vi "主画面.vi"() -> ()   [LabVIEW 2016]
uses:
  <vilib>/Utility/miscctls.llb/LVPointTypeDef.ctl
  <vilib>/ActorFramework/Message Enqueuer/Message Enqueuer.lvclass/Message Enqueuer.ctl
  <vilib>/Utility/miscctls.llb/LVRectTypeDef.ctl
  <vilib>/ActorFramework/Message Enqueuer/Enqueue.vi
  <vilib>/ActorFramework/Stop Msg/Stop Msg.lvclass
  C:/Program Files (x86)/National Instruments/LabVIEW 2016/vi.lib/ActorFramework/Message/Message.lvclass
  <vilib>/ActorFramework/Message Priority Queue/Priority Enqueue.vi
  data/FreeMem.dll
panel:
  out "运行时间":string="运行时间"
  out "ver":string
  out "权限等级 2":enum16{"一级权限", "二级权限", "三级权限", "超级权限"}(ring)
  out "权限等级":string
  out "布尔":bool
  in  "关于":bool
  out "SN":string="SN "
  in  "全屏":T1
  out "站点名称":string="站点名称"
  out "时间显示":string="2017-05-09 10:50:42"
  in  "主画面菜单":T2
  # "水质在线自动监测系统"
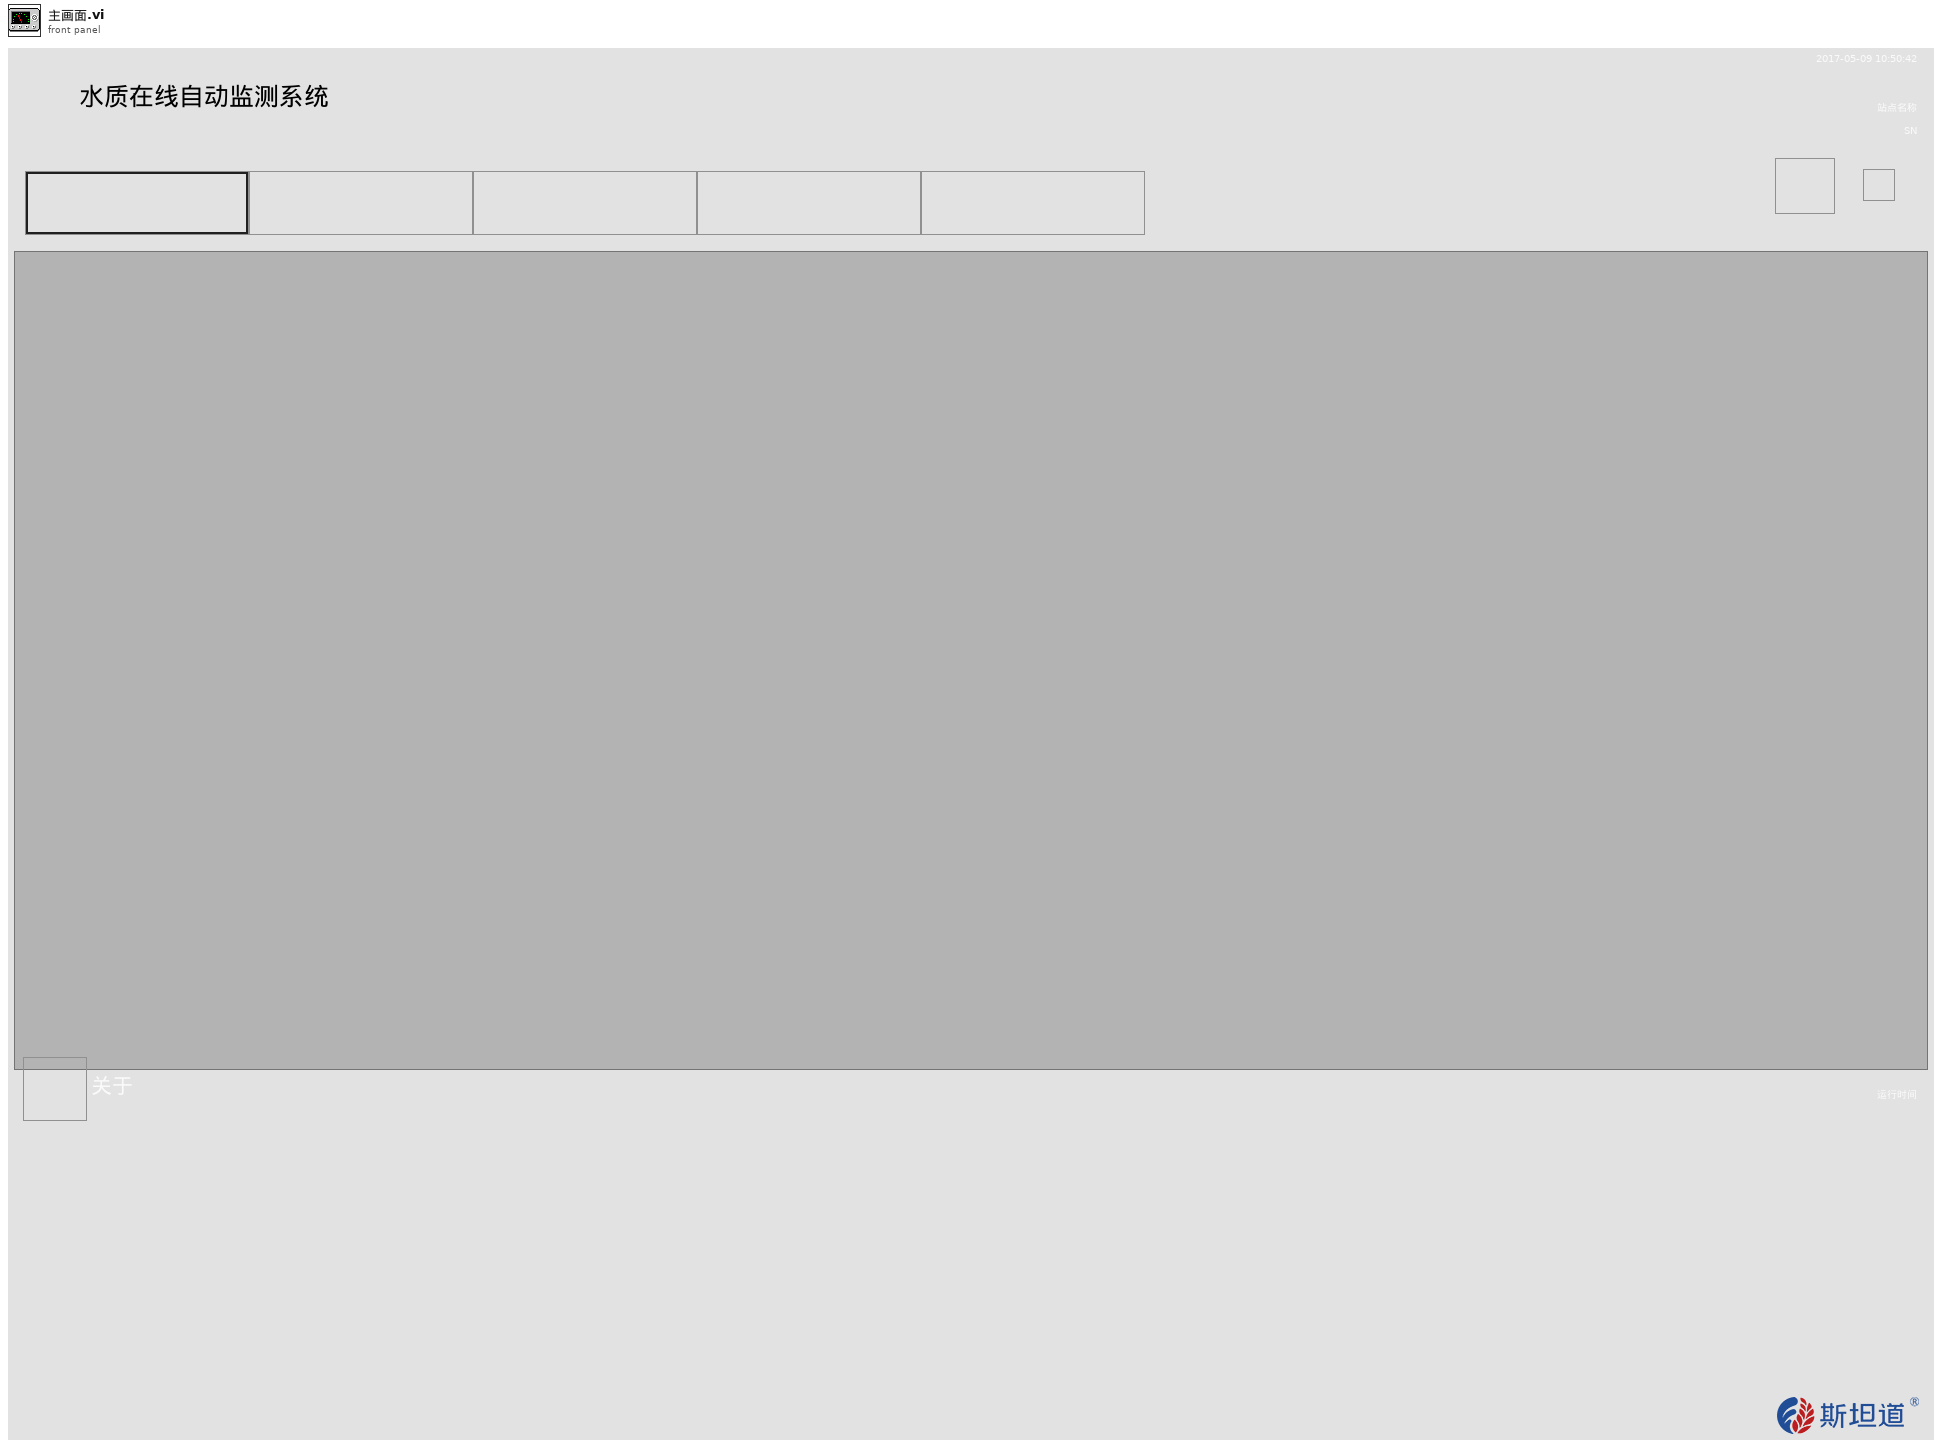
[diagram p1: front panel]
types:
  T1 = typedef "全屏按钮.ctl" = bool
  T2 = typedef "主画面单选控件.ctl" = enum32{"首页", "数据查询", "运维调试", "环境动力", "系统设置"}
  T3 = typedef "LVPointTypeDef.ctl" = cluster{"Horizontal":i16, "Vertical":i16}
  T4 = cluster{"时间标识":timestamp, "设备":string, "日志信息":string, "流程参数":string}
  T5 = enum32{"Bad", "Idle", "Run top level", "Running"}
  T6 = typedef "LVRectTypeDef.ctl" = cluster{"Left":i16, "Top":i16, "Right":i16, "Bottom":i16}
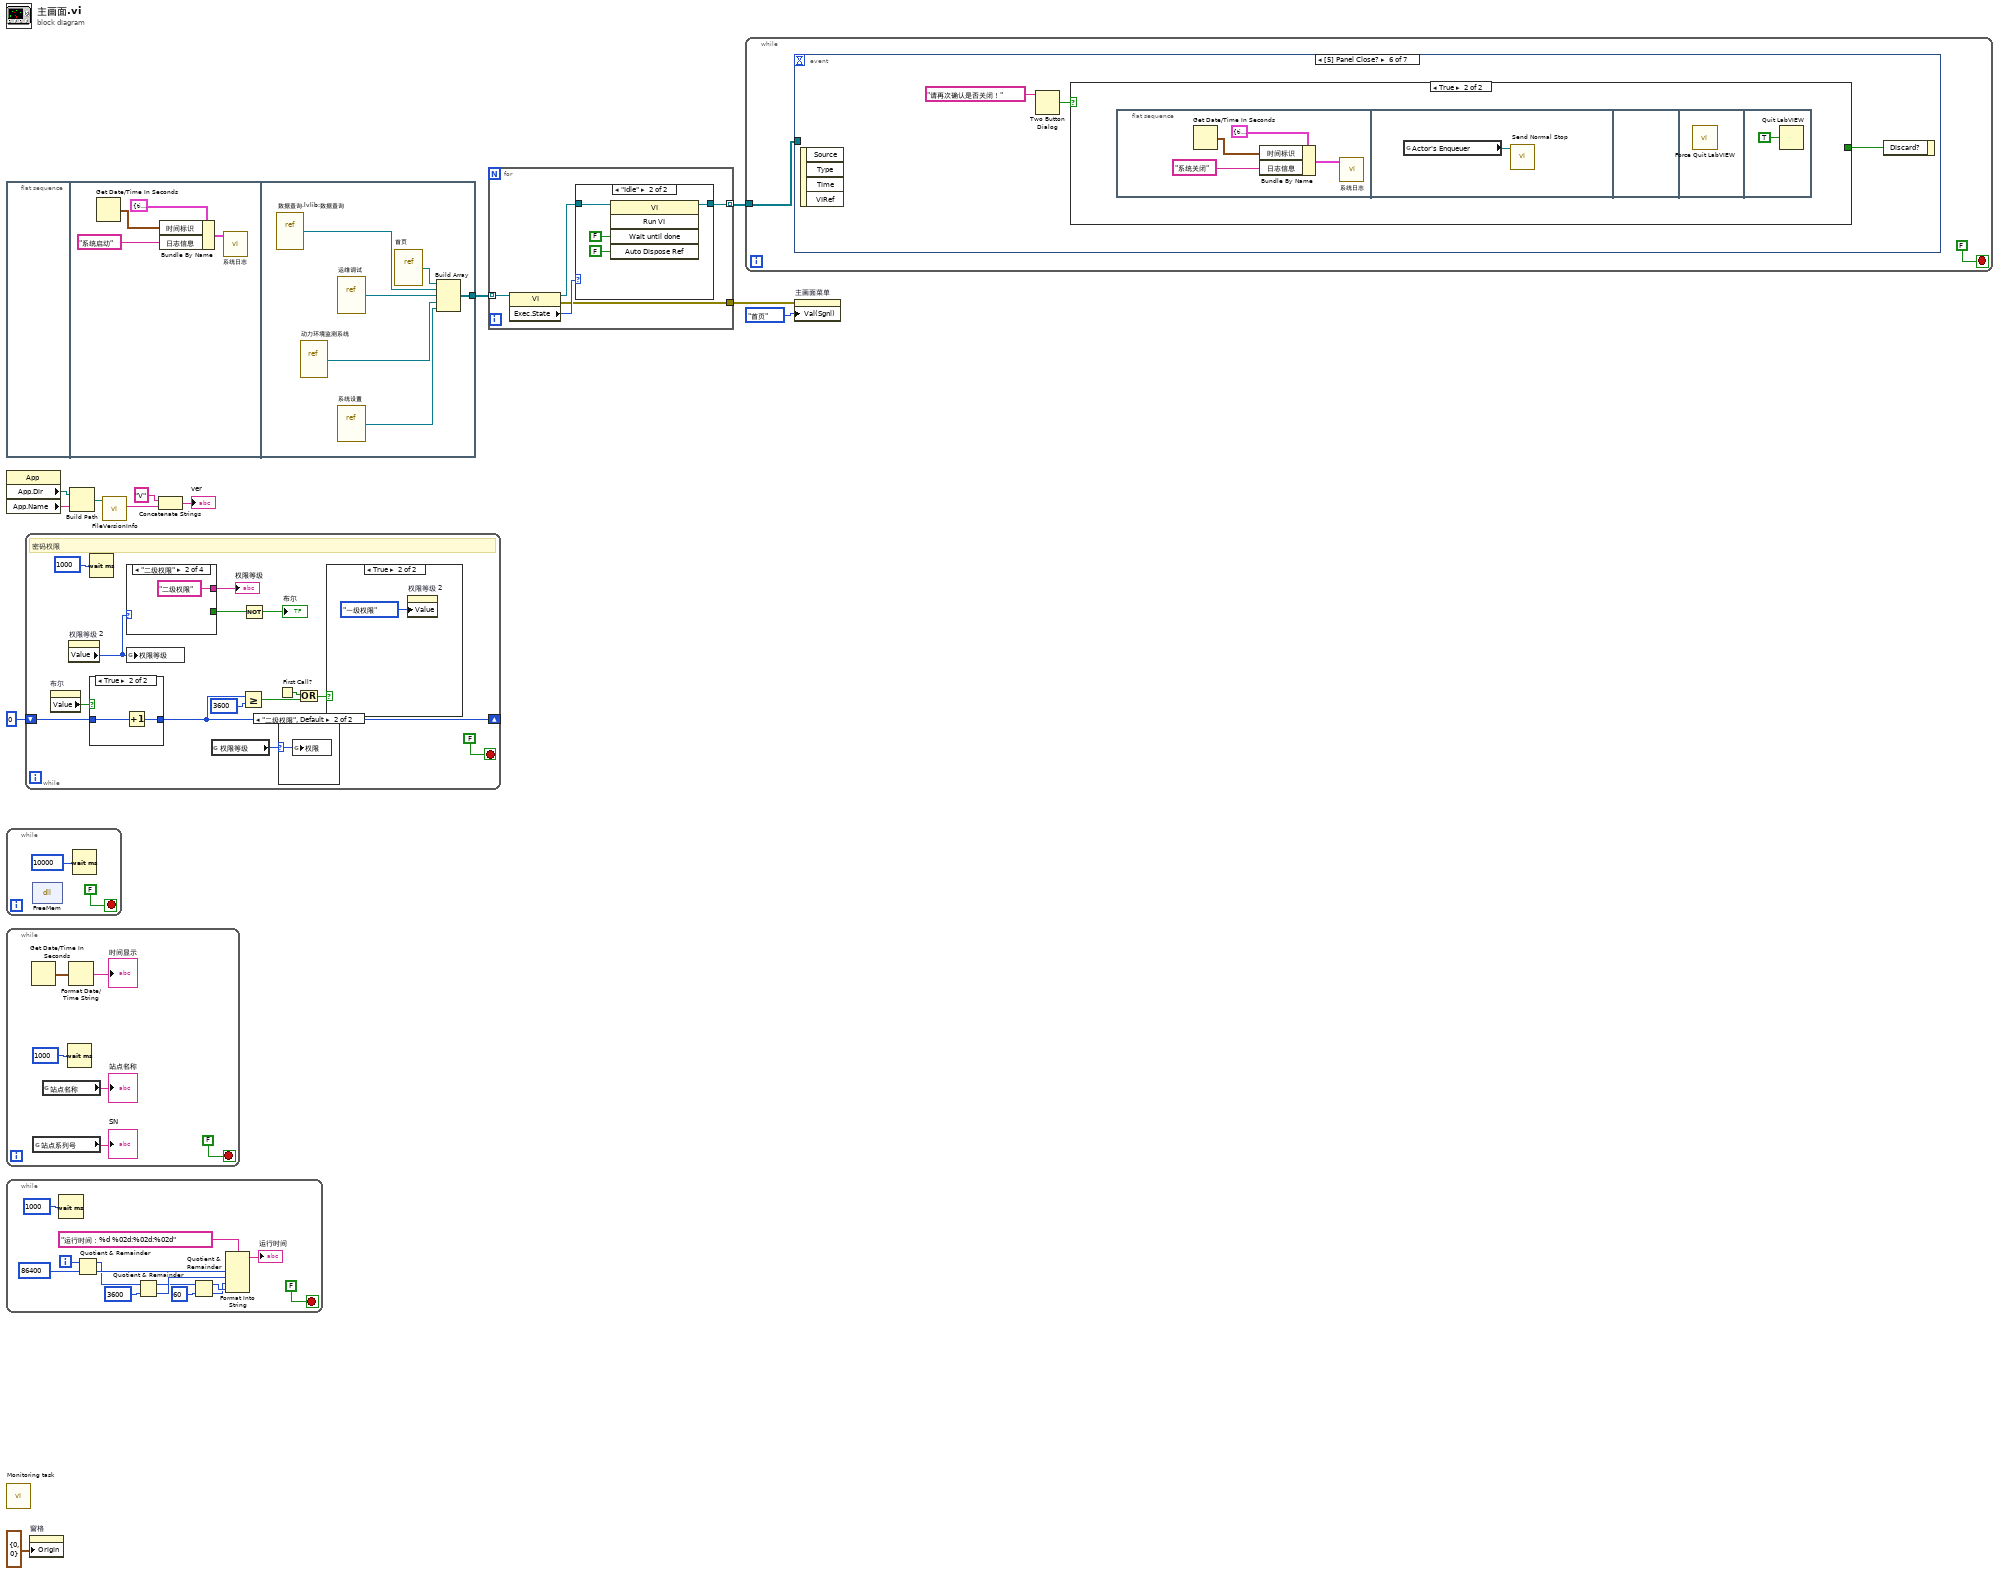
[diagram p0: block diagram]
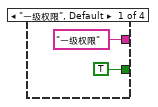
[diagram p3: hidden frame]
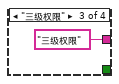
[diagram p4: hidden frame]
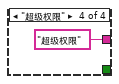
[diagram p5: hidden frame]
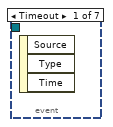
[diagram p9: hidden frame]
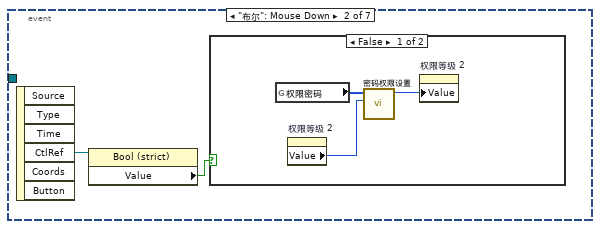
[diagram p10: hidden frame]
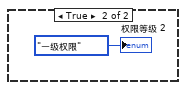
[diagram p11: hidden frame]
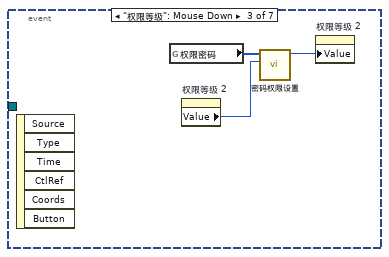
[diagram p12: hidden frame]
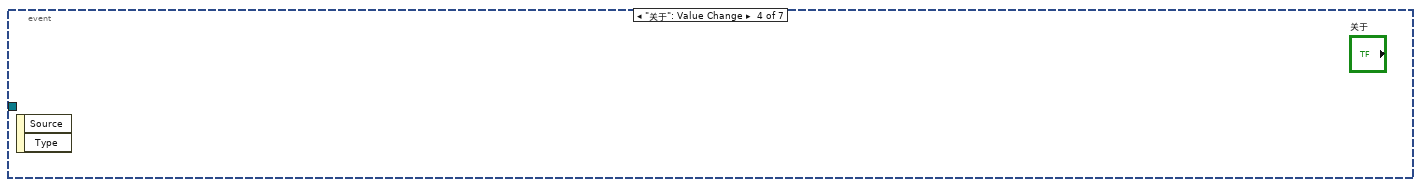
[diagram p13: hidden frame]
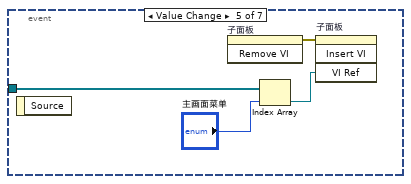
[diagram p14: hidden frame]
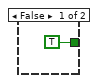
[diagram p15: hidden frame]
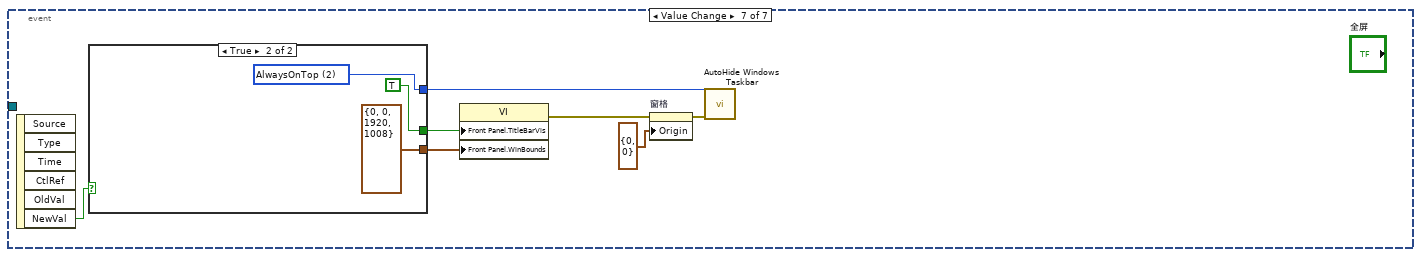
[diagram p16: hidden frame]
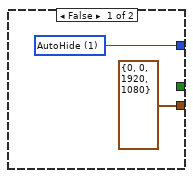
[diagram p17: hidden frame]
diagram:
  n1 = flat-sequence {
    tunnel: [w17] -> w10
    frame #0 {
    }
    frame #1 {
      n2 = Get Date/Time In Seconds() -> (seconds since 1Jan1904=w15:timestamp)
      n3 = Bundle By Name(cluster=T4 {"时间标识"=timestamp(0 s since 1904-01-01), "设备"="系统", "日志信息"="", "流程参数"=""} ("data in"), "时间标识"=w15, "日志信息"="系统启动") -> (w13:T4)
      n4 = call "系统日志.vi"("data in"=w13) -> ()  [unwired: 11 in]
    }
    frame #2 {
      n5 = vi-ref "数据查询.lvlib:数据查询.vi"() -> (w19:refnum<vi>)
      n6 = vi-ref "动力环境监测系统.vi"() -> (w22:refnum<vi>)
      n7 = vi-ref "运维调试.vi"() -> (w20:refnum<vi>)
      n8 = vi-ref "系统设置.vi"() -> (w21:refnum<vi>)
      n9 = vi-ref "首页.vi"() -> (w18:refnum<vi>)
      n10 = Build Array(w18, w19, w20, w22, w21) -> (w17:refnum<vi>[])
    }
  }
  n11 = property class="App"() -> ("App.Dir"=w6:path, "App.Name"=w4:string)  [unwired: 2 in, 2 out]
  n12 = while {
    stop <- FALSE stop-if-true
    n13 = dll-call lib="PTH2labs CUsersBin\tDocuments\nSourceCodeone-station-project-template多参数认证dataFreeMem.dll" fn="FreeMem"() -> ()  [unwired: 4 in, 2 out]
    n14 = Wait (ms)(milliseconds to wait=u32 10000 ("等待时间（毫秒）")) -> ()  [unwired: 1 out]
  }
  n15 = while {
    stop <- FALSE stop-if-true
    n16 = Get Date/Time In Seconds() -> (seconds since 1Jan1904=w27:timestamp)
    n17 = global read "系统设置全局变量.vi" "站点系列号"() -> (→"SN":string)
    n18 = global read "非断电保持全局变量.vi" "站点名称"() -> (→"站点名称":string)
    n19 = Wait (ms)(milliseconds to wait=u32 1000 ("等待时间（毫秒）")) -> ()  [unwired: 1 out]
    n20 = Format Date/Time String(seconds (now)=w27) -> (date/time string=→"时间显示":string)  [unwired: 2 in]
  }
  n21 = while {
    i -> [w32]
    stop <- FALSE stop-if-true
    n22 = Wait (ms)(milliseconds to wait=u32 1000 ("等待时间（毫秒）")) -> ()  [unwired: 1 out]
    n23 = Quotient & Remainder(x=w32, y=86400) -> (x-y*floor(x/y)=w34:i32, floor(x/y)=w40:i32)
    n24 = Quotient & Remainder(x=w34, y=3600) -> (x-y*floor(x/y)=w36:i32, floor(x/y)=w41:i32)
    n25 = Quotient & Remainder(x=w36, y=60) -> (x-y*floor(x/y)=w43:i32, floor(x/y)=w42:i32)
    n26 = Format Into String(format string="运行时间：%d %02d:%02d:%02d" ("格式字符串"), w40, w41, w42, w43) -> (resulting string=→"运行时间":string)  [unwired: 2 in, 1 out]
  }
  n27 = call "Monitoring task.vi"() -> ()  [unwired: 12 in]
  n28 = while {
    shift-right: [w55] -> _
    shift-left: u32 0 ("y") -> [w57]
    stop <- FALSE stop-if-true
    # "密码权限"
    n29 = property on="布尔" class="Bool (strict)"() -> ("Value"=w49:bool)  [unwired: 2 in, 2 out]
    n30 = property on="权限等级 2" class="Enum (strict)"() -> ("Value"=w46:enum16{"一级权限", "二级权限", "三级权限", "超级权限"})  [unwired: 2 in, 2 out]
    n31 = Wait (ms)(milliseconds to wait=u32 1000 ("等待时间（毫秒）")) -> ()  [unwired: 1 out]
    n32 = case shown="True" w49 {
      tunnel: w57 -> [_ w67]
      tunnel: [_ w66] -> w55
      frame False {
      }
      frame True {
        n33 = Increment(x=w67) -> (x+1=w66:u32)
      }
    }
    n34 = case shown="\"二级权限\"" w46 {
      tunnel: [TRUE _ _ _] -> w52
      tunnel: ["一级权限" "二级权限" "三级权限" "超级权限"] -> w51
      frame "一级权限", Default {
      }
      frame "二级权限" {
      }
      frame "三级权限" {
      }
      frame "超级权限" {
      }
    }
    "权限等级" <- w51
    n35 = global write "非断电保持全局变量.vi" "权限等级"(w46) -> ()
    n36 = global read "非断电保持全局变量.vi" "权限等级"() -> (w45:enum16{"一级权限", "二级权限", "三级权限", "超级权限"})
    n37 = Greater Or Equal?(x=w55, y=u32 3600) -> (x >= y?=w53:bool)
    n38 = Not(x=w52) -> (.not. x?=→"布尔":bool)
    n39 = First Call?() -> (First Call?: T/F=w47:bool)
    n40 = case shown="\"二级权限\", Default" w45 {
      selector: w45 -> [_ w59]
      frame "一级权限" {
      }
      frame "二级权限", Default {
        n41 = global write "多参数全局变量.vi" "权限"(w59) -> ()
      }
    }
    n42 = Or(x=w47, y=w53) -> (x .or. y?=w48:bool)
    n43 = case shown="True" w48 {
      frame False {
      }
      frame True {
        n44 = property on="权限等级 2" class="Enum (strict)"("Value"=enum16{"一级权限", "二级权限", "三级权限", "超级权限"}."一级权限" ("权限等级")) -> ()  [unwired: 2 in, 2 out]
      }
    }
  }
  n45 = property on="窗格" class="Pane"("Origin"=T3 {"Horizontal"=0, "Vertical"=0} ("原点")) -> ()  [unwired: 2 in, 2 out]
  n46 = Build Path(base path=w6, name or relative path=w4) -> (appended path=w5:path)
  n47 = call <vilib>:"FileVersionInfo.vi"("Application Path in"=w5) -> ("File Version Info"=w3:string)  [unwired: 7 in, 3 out]
  n48 = Concatenate Strings("V" ("字符串"), w3) -> (→"ver":string)
  n49 = for {
    tunnel: w10 -> [w72] mode=indexing
    tunnel: [w69] -> w7 mode=indexing
    tunnel: [w68] -> w8
    n50 = property class="VI"(reference=w72) -> (reference out=w70:refnum<vi>, error out=w68:errorcluster, "Exec.State"=w71:T5)  [unwired: 1 in]
    n51 = case shown="\"Idle\"" w71 {
      tunnel: w70 -> [w73 w75]
      tunnel: [w73 w74] -> w69
      frame "Bad", Default {
      }
      frame "Idle" {
        n52 = invoke class="VI" method="Run VI"(reference=w75, "Wait until done"=FALSE ("结束前等待"), "Auto Dispose Ref"=FALSE ("自动销毁引用")) -> (reference out=w74:refnum<vi>)  [unwired: 2 in, 4 out]
      }
    }
  }
  n53 = while {
    tunnel: w7 -> [w78]
    stop <- FALSE stop-if-true
    n54 = event shown="[5] Panel Close?" {
      selector: _ -> [_ _ _ _ _ _ _]
      dyn-events: _ -> [_ _ _ _ _ _ _]
      timeout: _ -> [_ _ _ _ _ _ _]
      tunnel: w78 -> [_ _ _ _ w89 _ _]
      event Timeout {
        n55 = event-data() -> ()  [unwired: 1 in, 3 out]
      }
      event "布尔": Mouse Down {
        n56 = event-data() -> ("CtlRef"=w81:refnum<vi>)  [unwired: 1 in, 5 out]
        n57 = property class="Bool (strict)"(reference=w81) -> ("Value"=w80:bool)  [unwired: 1 in, 2 out]
        n58 = case shown="False" w80 {
          frame False {
            n59 = global read "系统设置全局变量.vi" "权限密码"() -> (w84:u32[])
            n60 = property on="权限等级 2" class="Enum (strict)"() -> ("Value"=w82:enum16{"一级权限", "二级权限", "三级权限", "超级权限"})  [unwired: 2 in, 2 out]
            n61 = call "密码权限设置.vi"("权限输入"=w82, "权限密码"=w84) -> ("权限输出"=w83:enum16{"一级权限", "二级权限", "三级权限", "超级权限"})  [unwired: 9 in]
            n62 = property on="权限等级 2" class="Enum (strict)"("Value"=w83) -> ()  [unwired: 2 in, 2 out]
          }
          frame True {
            "权限等级 2" <- enum16{"一级权限", "二级权限", "三级权限", "超级权限"}."一级权限" ("权限等级")
          }
        }
      }
      event "权限等级": Mouse Down {
        n63 = event-data() -> ()  [unwired: 1 in, 6 out]
        n64 = global read "系统设置全局变量.vi" "权限密码"() -> (w88:u32[])
        n65 = property on="权限等级 2" class="Enum (strict)"() -> ("Value"=w87:enum16{"一级权限", "二级权限", "三级权限", "超级权限"})  [unwired: 2 in, 2 out]
        n66 = call "密码权限设置.vi"("权限输入"=w87, "权限密码"=w88) -> ("权限输出"=w86:enum16{"一级权限", "二级权限", "三级权限", "超级权限"})  [unwired: 9 in]
        n67 = property on="权限等级 2" class="Enum (strict)"("Value"=w86) -> ()  [unwired: 2 in, 2 out]
      }
      event "关于": Value Change {
        n68 = event-data() -> ()  [unwired: 1 in, 2 out]
      }
      event Value Change {
        n69 = event-data() -> ()  [unwired: 1 in, 1 out]
        n70 = invoke on="子面板" class="SubPnl" method="Remove VI"() -> (error out=w90:errorcluster)  [unwired: 3 in, 2 out]
        n71 = Index Array(array=w89, index="主画面菜单") -> (element=w91:refnum<vi>)
        n72 = invoke on="子面板" class="SubPnl" method="Insert VI"(error in=w90, "VI Ref"=w91) -> ()  [unwired: 2 in, 4 out]
      }
      event Panel Close? {
        n73 = event-data() -> ()  [unwired: 1 in, 4 out]
        n74 = Two Button Dialog(message="请再次确认是否关闭！" ("消息")) -> (T button?=w94:bool)  [unwired: 2 in]
        n75 = case shown="True" w94 {
          tunnel: [TRUE ("放弃？") _] -> w93
          frame False {
          }
          frame True {
            n76 = flat-sequence {
              frame #0 {
                n77 = Get Date/Time In Seconds() -> (seconds since 1Jan1904=w99:timestamp)
                n78 = Bundle By Name(cluster=T4 {"时间标识"=timestamp(0 s since 1904-01-01), "设备"="系统", "日志信息"="", "流程参数"=""} ("data in"), "时间标识"=w99, "日志信息"="系统关闭") -> (w97:T4)
                n79 = call "系统日志.vi"("data in"=w97) -> ()  [unwired: 11 in]
              }
              frame #1 {
                n80 = global read "工况数据接口全局.vi" "Actor's Enqueuer"() -> (w101:refnum<class "Message Enqueuer.lvclass">)
                n81 = call <vilib>:"Send Normal Stop.vi"("Message Enqueuer"=w101) -> ()  [unwired: 10 in, 1 out]
              }
              frame #2 {
              }
              frame #3 {
                n82 = call "Force Quit LabVIEW.vi"() -> ()  [unwired: 10 in, 2 out]
              }
              frame #4 {
                n83 = Quit LabVIEW(quit? (T)=TRUE ("退出？(T)")) -> ()
              }
            }
          }
        }
        n84 = event-data("Discard?"=w93) -> ()  [unwired: 1 in, 1 out]
      }
      event Value Change {
        n85 = event-data() -> ("NewVal"=w109:T1)  [unwired: 1 in, 5 out]
        n86 = case shown="True" w109 {
          tunnel: [w111 w114] -> w108
          tunnel: [T6 {"Left"=0, "Top"=0, "Right"=1920, "Bottom"=1080} ("前面板窗口:窗口边界") T6 {"Left"=0, "Top"=0, "Right"=1920, "Bottom"=1008} ("前面板窗口:窗口边界")] -> w103
          tunnel: [_ TRUE] -> w107
          frame False {
            w111 = u8 1 items=["AutoHide"=1, "AlwaysOnTop"=2] ("Operation")
          }
          frame True {
            w114 = u8 2 items=["AutoHide"=1, "AlwaysOnTop"=2] ("Operation")
          }
        }
        n87 = property class="VI"("Front Panel.TitleBarVis"=w107, "Front Panel.WinBounds"=w103) -> (error out=w105:errorcluster)  [unwired: 2 in, 1 out]
        n88 = property on="窗格" class="Pane"(error in=w105, "Origin"=T3 {"Horizontal"=0, "Vertical"=0} ("原点")) -> (error out=w104:errorcluster)  [unwired: 1 in, 1 out]
        n89 = call "AutoHide Windows Taskbar.vi"("error in (no error)"=w104, "Operation"=w108) -> ()  [unwired: 5 in, 1 out]
      }
    }
  }
  n90 = property on="主画面菜单" class="RadioBtnsControl (strict)"(error in=w8, "Val(Sgnl)"=主画面单选控件."首页" ("值(信号)")) -> ()  [unwired: 1 in, 2 out]
